vi "test substitute string.vi"() -> (2 "result":bool)   [LabVIEW 2019, in "ANODE Tests.lvlib"]
uses:
  ANODE Tests.lvlib
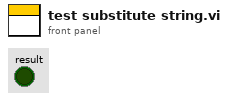
[diagram p1: front panel]
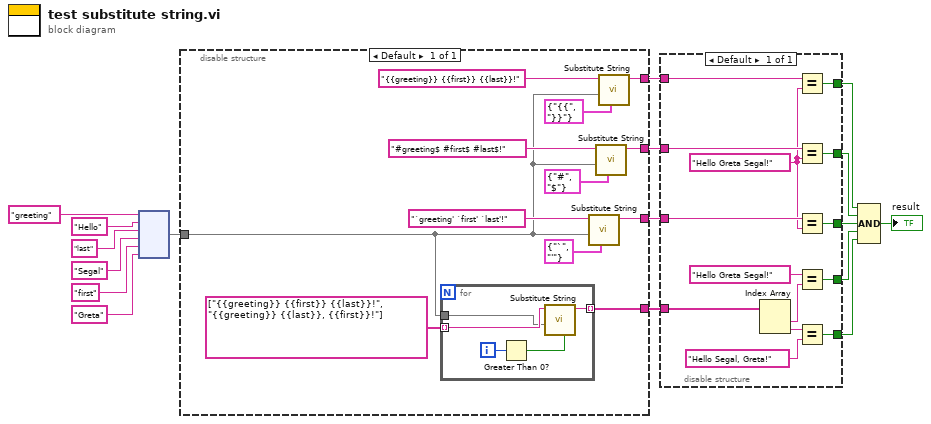
[diagram p0: block diagram]
diagram:
  n1 = node("greeting", "Hello", "last", "Segal", "first", "Greta") -> (w11:map{string, string})
  n2 = disable-structure shown="Default" {
    disable-tunnel: w11 -> [w19]
    disable-tunnel: [w23] -> w10
    disable-tunnel: [w22] -> w9
    disable-tunnel: [w21] -> w8
    disable-tunnel: [w18] -> w3
    frame Enabled {
      n3 = for {
        tunnel: string[] ["{{greeting}} {{first}} {{last}}!", "{{greeting}} {{last}}, {{first}}!"] -> [w34] mode=indexing
        tunnel: w19 -> [w33]
        tunnel: [w30] -> w18 mode=indexing
        i -> [w32]
        n4 = Greater Than 0?(x=w32) -> (x > 0?=w31:bool)
        n5 = call "Substitute String.vi"("use cached delimeter pattern data? (F)"=w31, "substitutions"=w33, "input string"=w34) -> ("output string"=w30:string)  [unwired: 7 in, 1 out]
      }
      n6 = call "Substitute String.vi"("delimeters"=cluster{"start":string, "end":string} {"start"="`", "end"="'"}, "substitutions"=w19, "input string"="`greeting' `first' `last'!" ("String in")) -> ("output string"=w23:string)  [unwired: 7 in, 1 out]
      n7 = call "Substitute String.vi"("delimeters"=cluster{"start":string, "end":string} {"start"="#", "end"="$"}, "substitutions"=w19, "input string"="#greeting$ #first$ #last$!" ("String in")) -> ("output string"=w22:string)  [unwired: 7 in, 1 out]
      n8 = call "Substitute String.vi"("delimeters"=cluster{"start":string, "end":string} {"start"="{{", "end"="}}"}, "substitutions"=w19, "input string"="{{greeting}} {{first}} {{last}}!" ("String in")) -> ("output string"=w21:string)  [unwired: 7 in, 1 out]
    }
  }
  n9 = disable-structure shown="Default" {
    disable-tunnel: w10 -> [w48]
    disable-tunnel: w9 -> [w47]
    disable-tunnel: w8 -> [w45]
    disable-tunnel: [w44] -> w7
    disable-tunnel: [w43] -> w6
    disable-tunnel: [w42] -> w5
    disable-tunnel: w3 -> [w41]
    disable-tunnel: [w39] -> w2
    disable-tunnel: [w35] -> w1
    frame Enabled {
      w46 = "Hello Greta Segal!" ("String out 3")
      n10 = Index Array(array=w41) -> (element #1=w38:string, element #2=w37:string)  [unwired: 2 in]
      n11 = Equal?(x=w45, y=w46) -> (x = y?=w44:bool)
      n12 = Equal?(x=w47, y=w46) -> (x = y?=w43:bool)
      n13 = Equal?(x=w48, y=w46) -> (x = y?=w42:bool)
      n14 = Equal?(x="Hello Greta Segal!" ("String out 3"), y=w38) -> (x = y?=w39:bool)
      n15 = Equal?(x=w37, y="Hello Segal, Greta!" ("String out 3")) -> (x = y?=w35:bool)
    }
  }
  n16 = Compound Arithmetic op=AND(w7, w6, w5, w2, w1) -> (→"result":bool)
